vi "STM32.DAC_sub_SineWaveCaculate.vi"(11 "频率":u16) -> (2 "调整后频率":u16, 3 "最优值":i32)   [LabVIEW 2012, in "Lib_UEL.ATE.lvlib" / "STM32-CoreBD.lvlib"]
uses:
  STM32-CoreBD.lvlib
panel:
  out "最优值结果":dbl
  out "运算数据":dbl[][](array[numeric])
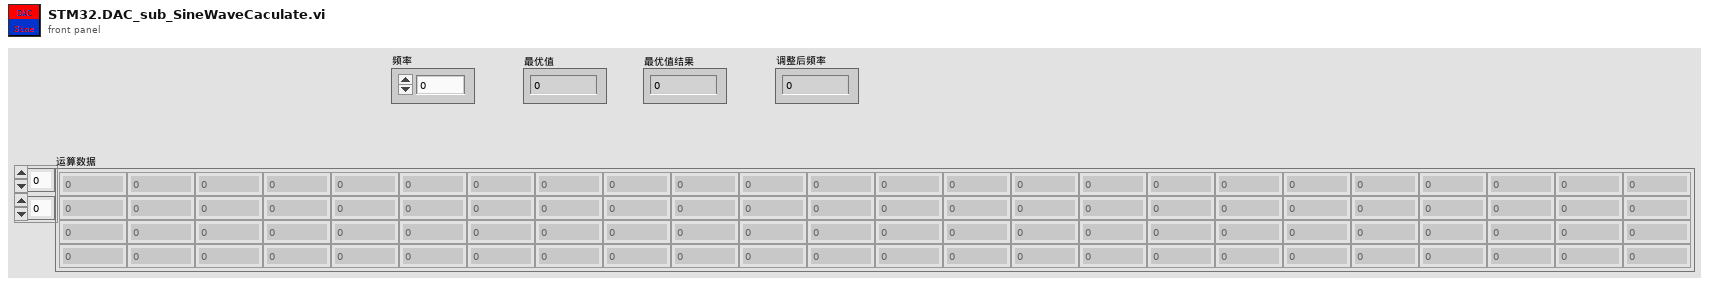
[diagram p1: front panel]
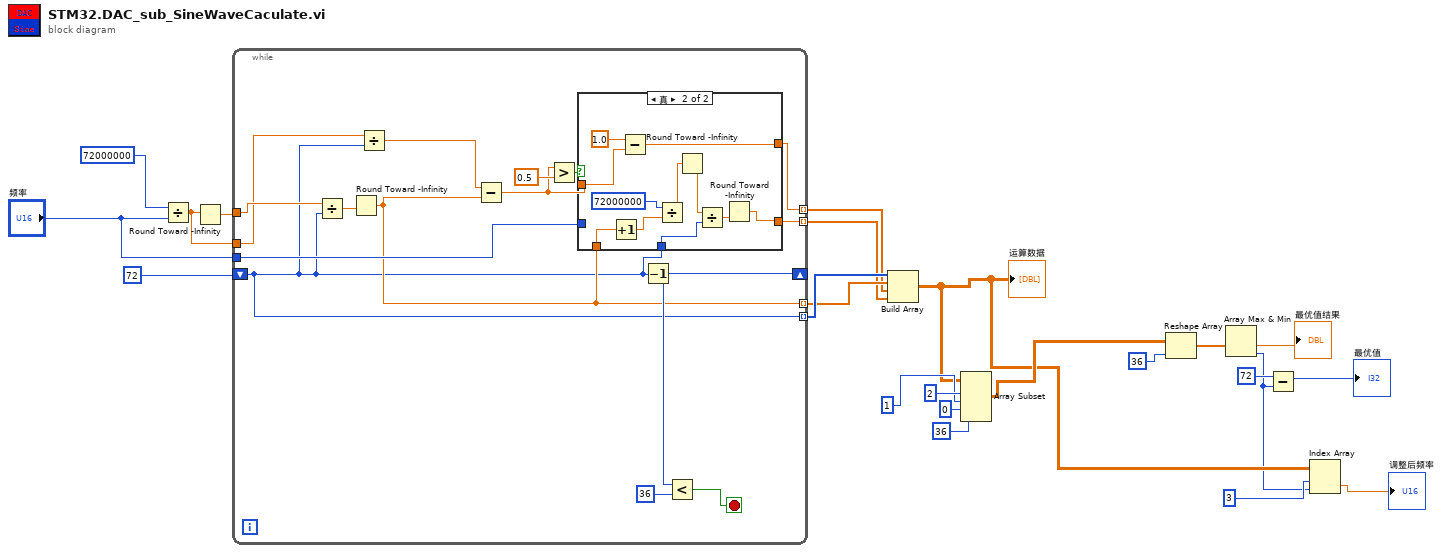
[diagram p0: block diagram]
diagram:
  n1 = Divide(x=72000000, y="频率") -> (x/y=w9:dbl)
  n2 = Round Toward -Infinity(1:w9) -> (0:w10:dbl)
  n3 = while {
    shift-right: [w36] -> _
    shift-left: 72 -> [w24]
    tunnel: w10 -> [w35]
    tunnel: [w28] -> w19 mode=indexing
    tunnel: [w25] -> w20 mode=indexing
    tunnel: [w24] -> w21 mode=indexing
    tunnel: w9 -> [w33]
    tunnel: [w26] -> w7 mode=indexing
    tunnel: "频率" -> [w27]
    stop <- w38 stop-if-true
    n4 = Divide(x=w35, y=w24) -> (x/y=w34:dbl)
    n5 = Round Toward -Infinity(1:w34) -> (0:w25:dbl)
    n6 = Divide(x=w33, y=w24) -> (x/y=w32:dbl)
    n7 = Subtract(x=w32, y=w25) -> (x-y=w29:dbl)
    n8 = Greater?(x=w29, y=0.5) -> (0:w30:bool)
    n9 = case shown="真" w30 {
      tunnel: w29 -> [w40 w50]
      tunnel: [w40 w49] -> w28
      tunnel: w27 -> [w39 _]
      tunnel: [w39 w43] -> w26
      tunnel: w25 -> [_ w42]
      tunnel: w24 -> [_ w47]
      frame False {
      }
      frame True {
        n10 = Increment(x=w42) -> (x+1=w41:dbl)
        n11 = Subtract(x=1.0, y=w50) -> (x-y=w49:dbl)
        n12 = Divide(x=72000000, y=w41) -> (x/y=w46:dbl)
        n13 = Round Toward -Infinity(1:w46) -> (0:w45:dbl)
        n14 = Divide(x=w45, y=w47) -> (x/y=w44:dbl)
        n15 = Round Toward -Infinity(1:w44) -> (0:w43:dbl)
      }
    }
    n16 = Decrement(x=w24) -> (x-1=w36:i32)
    n17 = Less?(x=w36, y=36) -> (x < y?=w38:bool)
  }
  n18 = Build Array(w21, w20, w19, w7) -> (w3:dbl[][])
  "运算数据" <- w3
  n19 = Array Subset(array=w3, index (row)=2 ("索引"), length (row)=1 ("长度"), index (col)=0 ("索引"), length (col)=36 ("长度")) -> (w6:dbl[][])
  n20 = Reshape Array(w6, 36 ("维数大小")) -> (w12:dbl[])
  n21 = Array Max & Min(array=w12) -> (min value=→"最优值结果":dbl, min index (indices)=w2:i32)  [unwired: 2 out]
  n22 = Subtract(x=72, y=w2) -> (x-y=→"最优值":i32)
  n23 = Index Array(array=w3, index (row)=3 ("禁用的索引 (列)"), index (col)=w2) -> (element=→"调整后频率":dbl)
